vi "VI Tree.vi"   [LabVIEW 2015, in "Ion Motion Roboclaw.lvlib"]
doc: "This is the instrument driver for the <INSTRUMENT NAME>. The VI Tree displays all the user-callable VIs of the instrument driver in an organized table."
uses:
  <instrlib>/Ion Motion Roboclaw/Ion Motion Roboclaw.lvlib
panel:
  # "(c) 2014 <Enter Company Name Here>.  ALL RIGHTS RESERVED."
  # "SEE DIAGRAM\nFOR VI TREE."
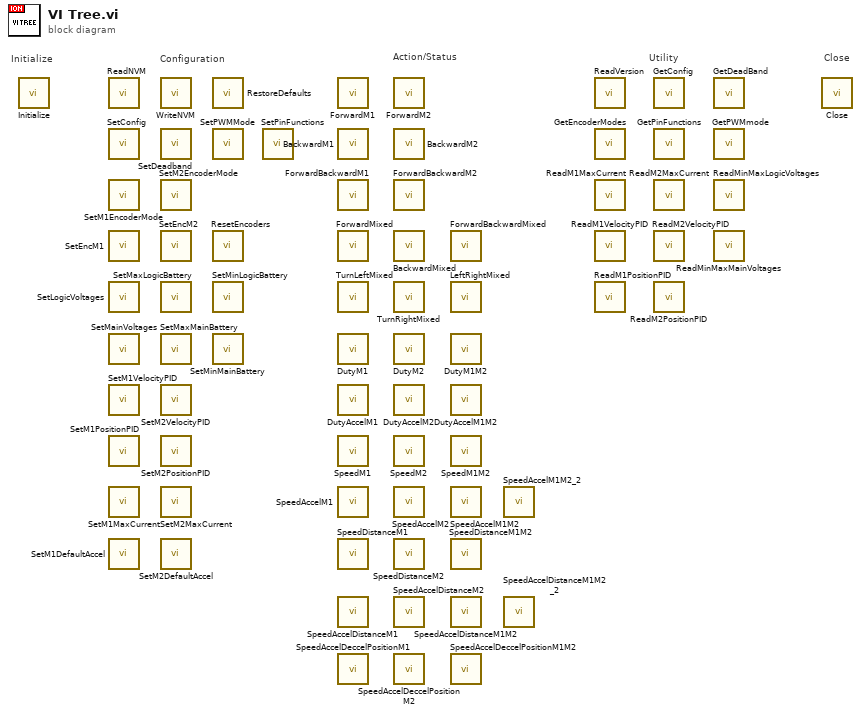
[diagram p0: block diagram]
diagram:
  # "Configuration"
  # "Utility"
  # "Action/Status"
  # "Close"
  # "Initialize"
  n1 = call <instrlib>:"Initialize.vi"() -> ()  [unwired: 10 in, 2 out]
  n2 = call <instrlib>:"ReadNVM.vi"() -> ()  [unwired: 9 in, 3 out]
  n3 = call <instrlib>:"SetConfig.vi"() -> ()  [unwired: 4 in, 3 out]
  n4 = call <instrlib>:"SetM1EncoderMode.vi"() -> ()  [unwired: 4 in, 3 out]
  n5 = call <instrlib>:"SetEncM1.vi"() -> ()  [unwired: 4 in, 3 out]
  n6 = call <instrlib>:"SetLogicVoltages.vi"() -> ()  [unwired: 6 in, 3 out]
  n7 = call <instrlib>:"SetMainVoltages.vi"() -> ()  [unwired: 6 in, 3 out]
  n8 = call <instrlib>:"SetM1VelocityPID.vi"() -> ()  [unwired: 13 in, 3 out]
  n9 = call <instrlib>:"SetM1PositionPID.vi"() -> ()  [unwired: 13 in, 3 out]
  n10 = call <instrlib>:"SetM1MaxCurrent.vi"() -> ()  [unwired: 4 in, 3 out]
  n11 = call <instrlib>:"SetM1DefaultAccel.vi"() -> ()  [unwired: 4 in, 3 out]
  n12 = call <instrlib>:"WriteNVM.vi"() -> ()  [unwired: 3 in, 3 out]
  n13 = call <instrlib>:"SetDeadband.vi"() -> ()  [unwired: 6 in, 3 out]
  n14 = call <instrlib>:"SetM2EncoderMode.vi"() -> ()  [unwired: 4 in, 3 out]
  n15 = call <instrlib>:"SetEncM2.vi"() -> ()  [unwired: 4 in, 3 out]
  n16 = call <instrlib>:"SetMaxLogicBattery.vi"() -> ()  [unwired: 4 in, 3 out]
  n17 = call <instrlib>:"SetMaxMainBattery.vi"() -> ()  [unwired: 4 in, 3 out]
  n18 = call <instrlib>:"SetM2VelocityPID.vi"() -> ()  [unwired: 13 in, 3 out]
  n19 = call <instrlib>:"SetM2PositionPID.vi"() -> ()  [unwired: 13 in, 3 out]
  n20 = call <instrlib>:"SetM2MaxCurrent.vi"() -> ()  [unwired: 4 in, 3 out]
  n21 = call <instrlib>:"SetM2DefaultAccel.vi"() -> ()  [unwired: 4 in, 3 out]
  n22 = call <instrlib>:"RestoreDefaults.vi"() -> ()  [unwired: 3 in, 3 out]
  n23 = call <instrlib>:"SetPWMMode.vi"() -> ()  [unwired: 4 in, 3 out]
  n24 = call <instrlib>:"ResetEncoders.vi"() -> ()  [unwired: 3 in, 3 out]
  n25 = call <instrlib>:"SetMinLogicBattery.vi"() -> ()  [unwired: 4 in, 3 out]
  n26 = call <instrlib>:"SetMinMainBattery.vi"() -> ()  [unwired: 4 in, 3 out]
  n27 = call <instrlib>:"SetPinFunctions.vi"() -> ()  [unwired: 6 in, 3 out]
  n28 = call <instrlib>:"ForwardM1.vi"() -> ()  [unwired: 4 in, 3 out]
  n29 = call <instrlib>:"BackwardM1.vi"() -> ()  [unwired: 4 in, 3 out]
  n30 = call <instrlib>:"ForwardBackwardM1.vi"() -> ()  [unwired: 4 in, 3 out]
  n31 = call <instrlib>:"ForwardMixed.vi"() -> ()  [unwired: 4 in, 3 out]
  n32 = call <instrlib>:"TurnLeftMixed.vi"() -> ()  [unwired: 4 in, 3 out]
  n33 = call <instrlib>:"DutyM1.vi"() -> ()  [unwired: 8 in, 3 out]
  n34 = call <instrlib>:"DutyAccelM1.vi"() -> ()  [unwired: 8 in, 3 out]
  n35 = call <instrlib>:"SpeedM1.vi"() -> ()  [unwired: 4 in, 3 out]
  n36 = call <instrlib>:"SpeedAccelM1.vi"() -> ()  [unwired: 6 in, 3 out]
  n37 = call <instrlib>:"SpeedDistanceM1.vi"() -> ()  [unwired: 6 in, 3 out]
  n38 = call <instrlib>:"SpeedAccelDistanceM1.vi"() -> ()  [unwired: 8 in, 3 out]
  n39 = call <instrlib>:"SpeedAccelDeccelPositionM1.vi"() -> ()  [unwired: 9 in, 3 out]
  n40 = call <instrlib>:"ForwardM2.vi"() -> ()  [unwired: 4 in, 3 out]
  n41 = call <instrlib>:"BackwardM2.vi"() -> ()  [unwired: 4 in, 3 out]
  n42 = call <instrlib>:"ForwardBackwardM2.vi"() -> ()  [unwired: 4 in, 3 out]
  n43 = call <instrlib>:"BackwardMixed.vi"() -> ()  [unwired: 4 in, 3 out]
  n44 = call <instrlib>:"TurnRightMixed.vi"() -> ()  [unwired: 4 in, 3 out]
  n45 = call <instrlib>:"DutyM2.vi"() -> ()  [unwired: 8 in, 3 out]
  n46 = call <instrlib>:"DutyAccelM2.vi"() -> ()  [unwired: 8 in, 3 out]
  n47 = call <instrlib>:"SpeedM2.vi"() -> ()  [unwired: 4 in, 3 out]
  n48 = call <instrlib>:"SpeedAccelM2.vi"() -> ()  [unwired: 6 in, 3 out]
  n49 = call <instrlib>:"SpeedDistanceM2.vi"() -> ()  [unwired: 6 in, 3 out]
  n50 = call <instrlib>:"SpeedAccelDistanceM2.vi"() -> ()  [unwired: 8 in, 3 out]
  n51 = call <instrlib>:"SpeedAccelDeccelPositionM2.vi"() -> ()  [unwired: 9 in, 3 out]
  n52 = call <instrlib>:"ForwardBackwardMixed.vi"() -> ()  [unwired: 4 in, 3 out]
  n53 = call <instrlib>:"LeftRightMixed.vi"() -> ()  [unwired: 4 in, 3 out]
  n54 = call <instrlib>:"DutyM1M2.vi"() -> ()  [unwired: 8 in, 3 out]
  n55 = call <instrlib>:"DutyAccelM1M2.vi"() -> ()  [unwired: 8 in, 3 out]
  n56 = call <instrlib>:"SpeedM1M2.vi"() -> ()  [unwired: 6 in, 3 out]
  n57 = call <instrlib>:"SpeedAccelM1M2.vi"() -> ()  [unwired: 6 in, 3 out]
  n58 = call <instrlib>:"SpeedDistanceM1M2.vi"() -> ()  [unwired: 9 in, 3 out]
  n59 = call <instrlib>:"SpeedAccelDistanceM1M2.vi"() -> ()  [unwired: 9 in, 3 out]
  n60 = call <instrlib>:"SpeedAccelDeccelPositionM1M2.vi"() -> ()  [unwired: 17 in, 3 out]
  n61 = call <instrlib>:"SpeedAccelM1M2_2.vi"() -> ()  [unwired: 8 in, 3 out]
  n62 = call <instrlib>:"SpeedAccelDistanceM1M2_2.vi"() -> ()  [unwired: 13 in, 3 out]
  n63 = call <instrlib>:"ReadVersion.vi"() -> ()  [unwired: 5 in, 4 out]
  n64 = call <instrlib>:"GetEncoderModes.vi"() -> ()  [unwired: 6 in, 5 out]
  n65 = call <instrlib>:"ReadM1MaxCurrent.vi"() -> ()  [unwired: 5 in, 4 out]
  n66 = call <instrlib>:"ReadM1VelocityPID.vi"() -> ()  [unwired: 5 in, 4 out]
  n67 = call <instrlib>:"ReadM1PositionPID.vi"() -> ()  [unwired: 5 in, 4 out]
  n68 = call <instrlib>:"GetConfig.vi"() -> ()  [unwired: 5 in, 4 out]
  n69 = call <instrlib>:"GetPinFunctions.vi"() -> ()  [unwired: 5 in, 4 out]
  n70 = call <instrlib>:"ReadM2MaxCurrent.vi"() -> ()  [unwired: 5 in, 4 out]
  n71 = call <instrlib>:"ReadM2VelocityPID.vi"() -> ()  [unwired: 5 in, 4 out]
  n72 = call <instrlib>:"ReadM2PositionPID.vi"() -> ()  [unwired: 5 in, 4 out]
  n73 = call <instrlib>:"GetDeadBand.vi"() -> ()  [unwired: 6 in, 5 out]
  n74 = call <instrlib>:"GetPWMmode.vi"() -> ()  [unwired: 5 in, 4 out]
  n75 = call <instrlib>:"ReadMinMaxLogicVoltages.vi"() -> ()  [unwired: 7 in, 4 out]
  n76 = call <instrlib>:"ReadMinMaxMainVoltages.vi"() -> ()  [unwired: 6 in, 5 out]
  n77 = call <instrlib>:"Close.vi"() -> ()  [unwired: 11 in, 1 out]
